vi "Write Enable TLS_.vi"(8 "error in (no error)":errorcluster, 10 "Enable TLS?":bool, 11 "TCPSocketBasedCommHandlerBase in":refnum<class "TCPSocketBasedCommHandlerBase.lvclass">) -> (0 "error out":errorcluster, 3 "TCPSocketBasedCommHandlerBase out":refnum<class "TCPSocketBasedCommHandlerBase.lvclass">)   [LabVIEW 2020, in "wamplv.lvlib" / "TCPSocketBasedCommHandlerBase.lvclass"]
uses:
  TCPSocketBasedCommHandlerBase.lvclass
  TCPSocketBasedCommHandlerBase.lvclass/TCPSocketBasedCommHandlerBase.ctl
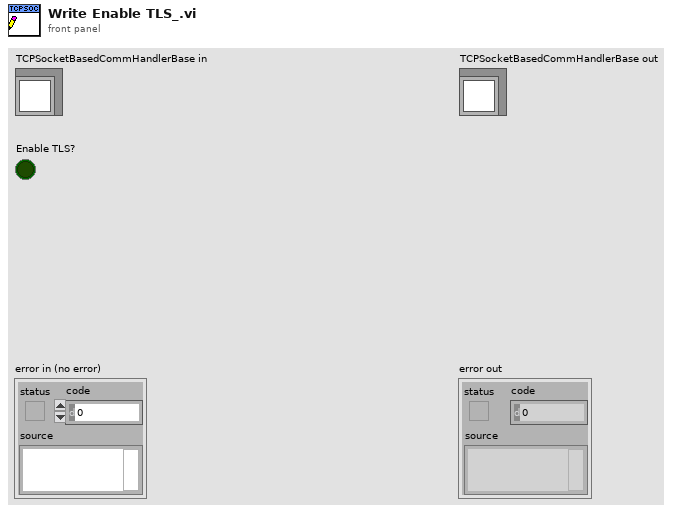
[diagram p1: front panel]
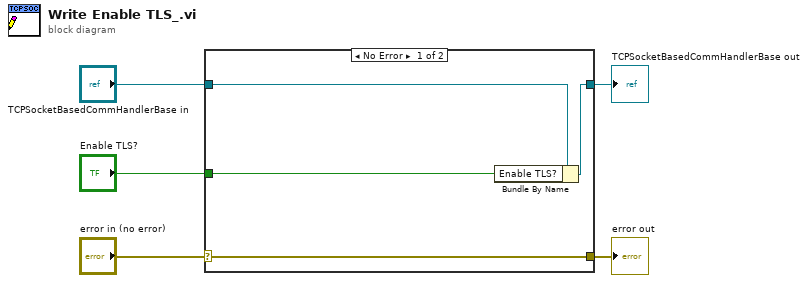
[diagram p0: block diagram]
diagram:
  n1 = case shown="No Error" "error in (no error)" {
    selector: "error in (no error)" -> [w9 w10]
    tunnel: [w9 w10] -> w4
    tunnel: [w7 w11] -> w2
    tunnel: "TCPSocketBasedCommHandlerBase in" -> [w8 w11]
    tunnel: "Enable TLS?" -> [w6 _]
    frame No Error {
      n2 = Bundle By Name(cluster=w8, "Enable TLS?"=w6) -> (w7:refnum<class "TCPSocketBasedCommHandlerBase.lvclass">)
    }
    frame Error {
    }
  }
  "error out" <- w4
  "TCPSocketBasedCommHandlerBase out" <- w2
